vi "Part 2.vi"(11 "Input":string) -> (3 "Output":i64)   [LabVIEW 2021]
uses:
  9d18ff97-46f7-4c5e-b407-81b26697cff8.vi
panel:
  out "Array":bool[][](array[boolean])
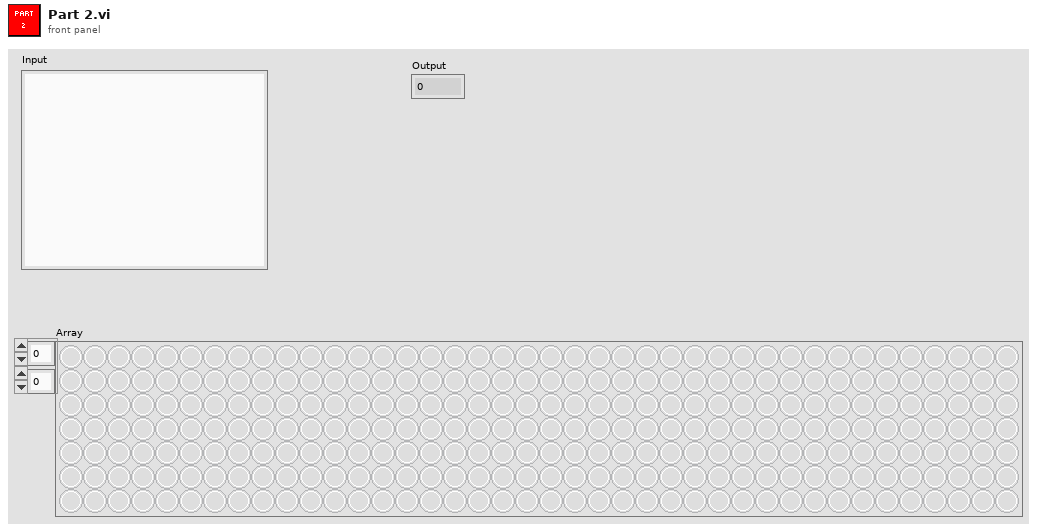
[diagram p1: front panel]
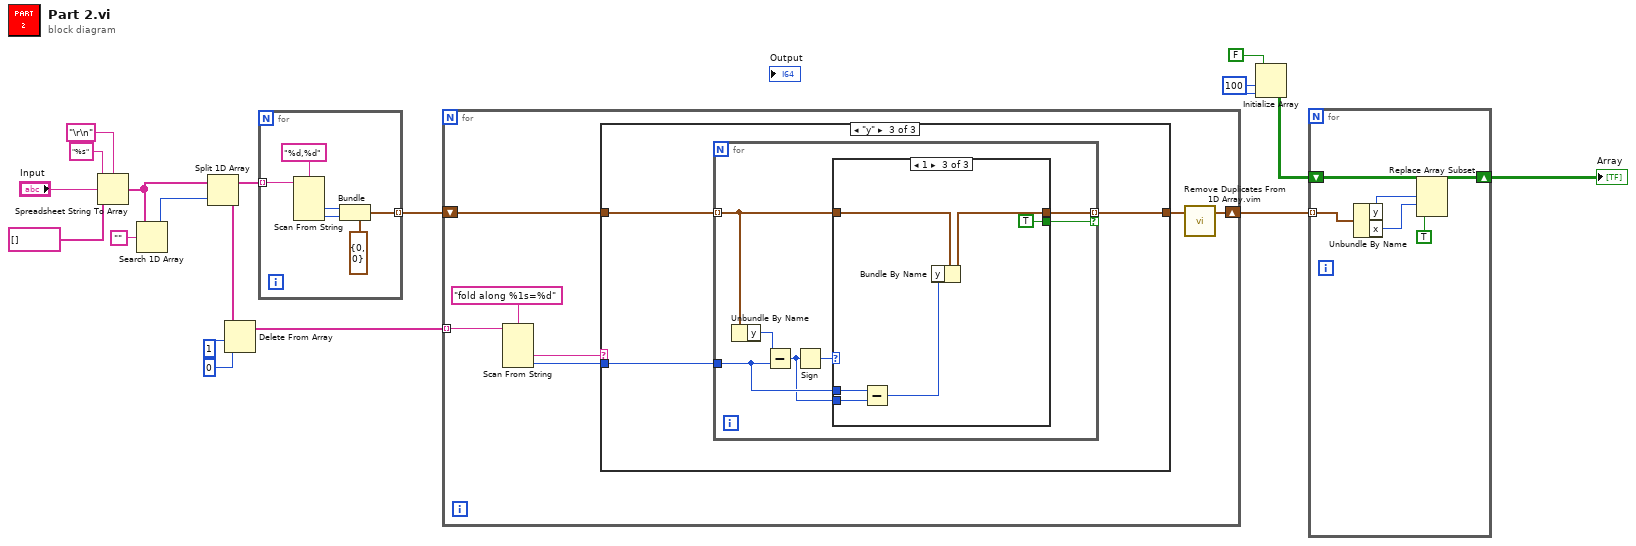
[diagram p0: block diagram]
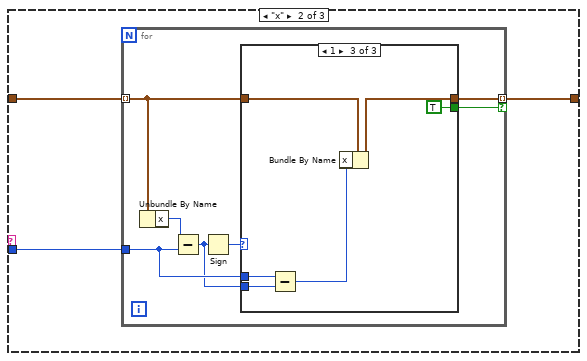
[diagram p3: hidden frame]
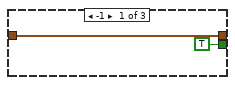
[diagram p4: hidden frame]
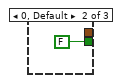
[diagram p5: hidden frame]
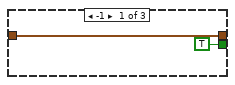
[diagram p6: hidden frame]
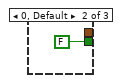
[diagram p7: hidden frame]
diagram:
  w4 = 100 ("dimension size")
  n1 = Spreadsheet String To Array(delimiter (Tab)="\r\n", format string="%s", spreadsheet string="Input", array type (2D Dbl)=string[] []) -> (array=w14:string[])
  n2 = Search 1D Array(1D array=w14, element="") -> (index of element=w13:i32)  [unwired: 1 in]
  n3 = Split 1D Array(array=w14, index=w13) -> (first subarray=w8:string[], second subarray=w9:string[])
  n4 = Delete From Array(array=w9, length=1 ("index"), index=0) -> (array with subset deleted=w10:string[])  [unwired: 1 out]
  n5 = for {
    tunnel: w8 -> [w24] mode=indexing
    tunnel: [w21] -> w7 mode=indexing
    n6 = Scan From String(format string="%d,%d", input string=w24) -> (output 1=w22:i32, output 2=w20:i32)  [unwired: 4 in, 3 out]
    n7 = Bundle(cluster=cluster{"x":i32, "y":i32} {"x"=0, "y"=0}, "x"=w22, "y"=w20) -> (w21:cluster{"x":i32, "y":i32})
  }
  n8 = for {
    tunnel: w10 -> [w31] mode=indexing
    shift-right: [w25] -> w5
    shift-left: w7 -> [w27]
    n9 = Scan From String(format string="fold along %1s=%d", input string=w31) -> (output 1=w29:string, output 2=w28:i32)  [unwired: 4 in, 3 out]
    n10 = case shown="\"y\"" w29 {
      tunnel: w28 -> [_ w35 w54]
      tunnel: w27 -> [w32 w34 w53]
      tunnel: [w32 w33 w52] -> w26
      frame Default {
      }
      frame "x" {
        n11 = for {
          tunnel: w34 -> [w40] mode=indexing
          tunnel: w35 -> [w37]
          tunnel: [w39] -> w33 mode=indexing if=w38
          n12 = Unbundle By Name(w40) -> ("x"=w41:i32)
          n13 = Subtract(x=w41, y=w37) -> (x-y=w36:i32)
          n14 = Sign(1:w36) -> (0:w42:i32)
          n15 = case shown="1" w42 {
            tunnel: [w44 _ w49] -> w39
            tunnel: w40 -> [w44 _ w50]
            tunnel: [TRUE FALSE TRUE] -> w38
            tunnel: w37 -> [_ _ w48]
            tunnel: w36 -> [_ _ w47]
            frame -1 {
            }
            frame 0, Default {
            }
            frame 1 {
              n16 = Subtract(x=w48, y=w47) -> (x-y=w46:i32)
              n17 = Bundle By Name(cluster=w50, "x"=w46) -> (w49:cluster{"x":i32, "y":i32})
            }
          }
        }
      }
      frame "y" {
        n18 = for {
          tunnel: w53 -> [w59] mode=indexing
          tunnel: w54 -> [w56]
          tunnel: [w58] -> w52 mode=indexing if=w57
          n19 = Unbundle By Name(w59) -> ("y"=w60:i32)
          n20 = Subtract(x=w60, y=w56) -> (x-y=w55:i32)
          n21 = Sign(1:w55) -> (0:w61:i32)
          n22 = case shown="1" w61 {
            tunnel: [w63 _ w68] -> w58
            tunnel: w59 -> [w63 _ w69]
            tunnel: [TRUE FALSE TRUE] -> w57
            tunnel: w56 -> [_ _ w67]
            tunnel: w55 -> [_ _ w66]
            frame -1 {
            }
            frame 0, Default {
            }
            frame 1 {
              n23 = Subtract(x=w67, y=w66) -> (x-y=w65:i32)
              n24 = Bundle By Name(cluster=w69, "y"=w65) -> (w68:cluster{"x":i32, "y":i32})
            }
          }
        }
      }
    }
    n25 = call "Remove Duplicates From 1D Array.vim"("array"=w26) -> ("array with duplicates removed"=w25:cluster{"x":i32, "y":i32}[])  [unwired: 10 in]
  }
  n26 = Initialize Array(FALSE, w4, w4) -> (w2:bool[][])
  n27 = for {
    tunnel: w5 -> [w74] mode=indexing
    shift-right: [w75] -> w1
    shift-left: w2 -> [w76]
    n28 = Unbundle By Name(w74) -> ("y"=w73:i32, "x"=w72:i32)
    n29 = Replace Array Subset(array=w76, new element=TRUE, index (row)=w73, index (col)=w72) -> (w75:bool[][])
  }
  "Array" <- w1
